vi "adapter_rm_depth_ahat.vi"(10 "configuration_rm_depth_ahat":T1={"chunk"=4096, "mode"=1, "divisor"=1, "profile_z"=0, "profile_ab"=3, "level"=255, "_reserved_0"=0, "_reserved_1"=0, "_reserved_2"=0, "bitrate"=0, "_reserved_3"=0, "options_size"=-1, "options_data"=0, "_reserved_4"=0}, 11 "path in":path=path "hl2ss_ulm.dll") -> (2 "configuration":u64, 3 "path out":path)   [LabVIEW 2023]
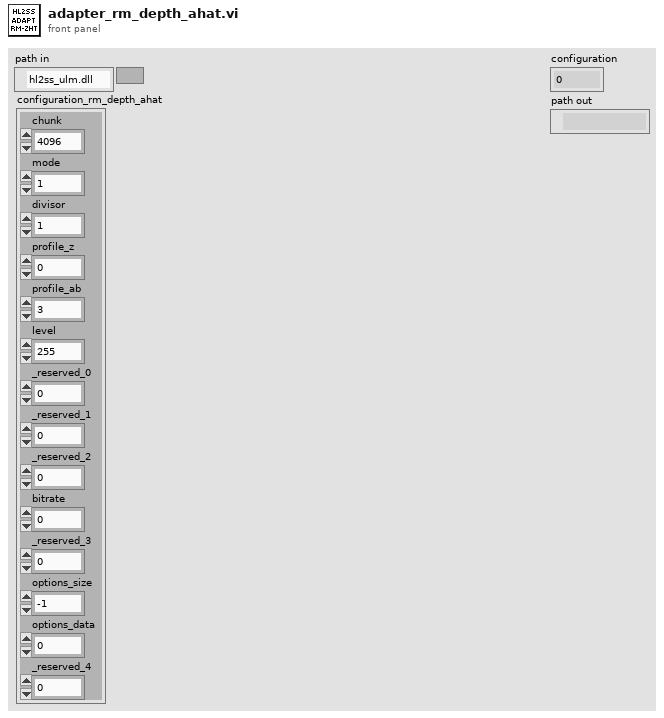
[diagram p1: front panel]
types:
  T1 = cluster{"chunk":u64, "mode":u8, "divisor":u8, "profile_z":u8, "profile_ab":u8, "level":u8, "_reserved_0":u8, "_reserved_1":u8, "_reserved_2":u8, "bitrate":u32, "_reserved_3":u32, "options_size":i64, "options_data":u64, "_reserved_4":u64}
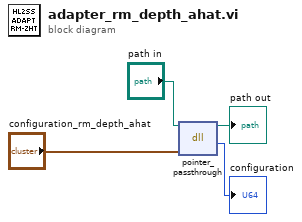
[diagram p0: block diagram]
diagram:
  n1 = dll-call lib="C:/Users/jcds/Documents/GitHub/hl2ss/extensions/client_labview/hl2ss_ulm.dll" fn="pointer_passthrough"(path in="path in", "p"="configuration_rm_depth_ahat") -> (path out=→"path out":path, "return type"=→"configuration":u64)  [unwired: 3 in, 1 out]
